vi "Read Elevator Call.vi"(8 "error in (no error)":errorcluster, 11 "User Console in":refnum<class "User Console.lvclass">) -> (0 "error out":errorcluster, 2 "Elevator Call":T1, 3 "User Console out":refnum<class "User Console.lvclass">)   [LabVIEW 2019, in "User Console Actor.lvlib" / "User Console.lvclass"]
uses:
  User Console.lvclass
  Elevator Call.ctl
  User Console.lvclass/User Console.ctl
  Abstract User Console Actor/Abstract User Console Actor/Abstract User Console.lvclass
panel:
  # "Fourth Floor"
  # "Third Floor"
  # "Second Floor"
  # "First Floor"
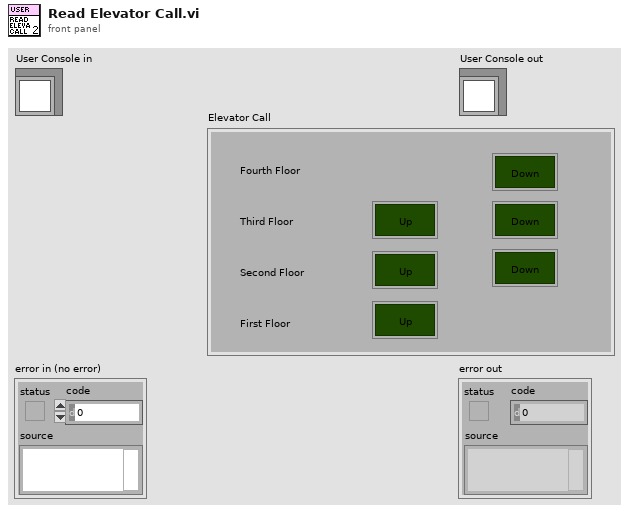
[diagram p1: front panel]
types:
  T1 = typedef "User Console Actor.lvlib/User Console.lvclass/Elevator Call.ctl" = cluster{"Up":bool, "Up 2":bool, "Up 3":bool, "Down":bool, "Down 2":bool, "Down 3":bool}
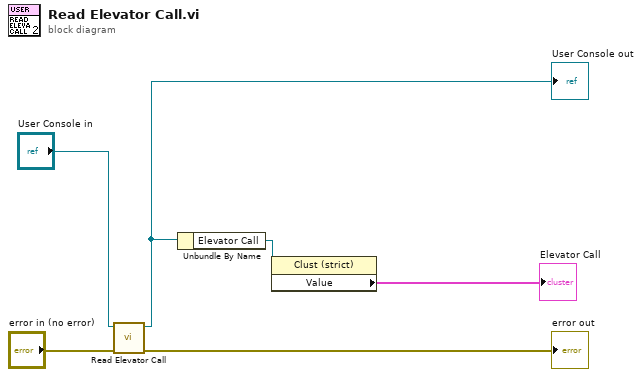
[diagram p0: block diagram]
diagram:
  n1 = call-parent "Read Elevator Call.vi"("error in (no error)"="error in (no error)", "Abstract User Console in"="User Console in") -> ("error out"=→"error out":errorcluster, "Abstract User Console out"=w3:refnum<class "User Console.lvclass">)  [unwired: 7 in, 1 out]
  "User Console out" <- w3
  n2 = Unbundle By Name(w3) -> ("Elevator Call"=w2:refnum<vi>)
  n3 = property class="Clust (strict)"(reference=w2) -> ("Value"=→"Elevator Call":T1)  [unwired: 1 in, 2 out]
